vi "Convert to String.vi"(11 "keyed array":T1) -> (3 "KA string":string)   [LabVIEW 2015, in "Car Wash.lvlib" / "Tools_KeyedArray.lvlib"]
uses:
  Tools_KeyedArray.lvlib
  KeyedArray.ctl
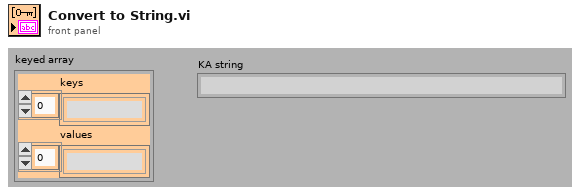
[diagram p1: front panel]
types:
  T1 = typedef "Car Wash.lvlib/Tools_KeyedArray.lvlib/KeyedArray.ctl" = cluster{"keys":string[], "values":string[]}
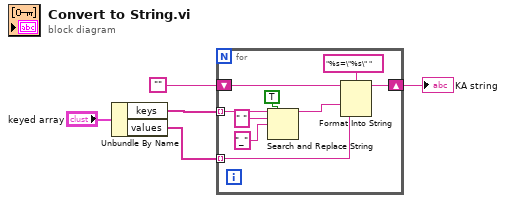
[diagram p0: block diagram]
diagram:
  n1 = Unbundle By Name("keyed array") -> ("keys"=w4:string[], "values"=w5:string[])
  n2 = for {
    tunnel: w4 -> [w10] mode=indexing
    tunnel: w5 -> [w12] mode=indexing
    shift-right: [w13] -> w3
    shift-left: "" -> [w14]
    n3 = Search and Replace String(replace all?=TRUE ("replace all? (F)"), input string=w10, search string=" ", replace string="_" ("replace string (\"\")")) -> (result string=w9:string)  [unwired: 1 in, 6 out]
    n4 = Format Into String(format string="%s=\"%s\" ", initial string=w14, w9, w12) -> (resulting string=w13:string)  [unwired: 1 in, 1 out]
  }
  "KA string" <- w3
